vi "Compile ESTTL.vi"(8 "error in (no error)":errorcluster, 10 "PB-01 Compiled Data":T1, 11 "Device Item Ref in":T4 format="%.0x") -> (0 "error out":errorcluster, 2 "PB-01 Compiled Data out":T1, 3 "Device Item Ref out":T4 format="%.0x")   [LabVIEW 2015, in "DCM System Explorer.lvlib"]
uses:
  DCM System Explorer.lvlib
  <vilib>/NI Veristand/Custom Device API/Custom Device Item Ref.ctl
  Shared/Types/ESTTL Setup Indexes.ctl
  Shared/Types/PB-01.ctl
  <vilib>/Powertrain Controls/Device Drivers/VR-Hall/RevC/Real-Time/Support/Vr_Hall_mode_control_revc.ctl
  Shared/DCM Constants and GUIDs.vi
  <vilib>/NI Veristand/Custom Device Tools/Custom Device Utility Library/NI VeriStand - Search for Item by GUID.vi
  <vilib>/NI Veristand/Custom Device Tools/Custom Device Utility Library/Custom Device Utility Library.lvlib
  DCM Shared.lvlib
  <vilib>/NI VeriStand/Custom Device API/Custom Device API.lvlib
panel:
  in  "Command":T2[](array[typedef])=[{"Mode"=-1, "Polarity"=-1, "Frequency [Hz]"=-1, "Duty Cycle [%]"=-1, "TDC Offset [CAD]"=-1, "Window Start [DBTDC]"=-1, "Window End [DBTDC]"=0, "Angles"=[{"Enable"=0, "Location [DBTDC]"=0, "Duration [s]"=0}, {"Enable"=0, "Location [DBTDC]"=0, "Duration [s]"=0}, {"Enable"=0, "Location [DBTDC]"=0, "Duration [s]"=0}, {"Enable"=0, "Location [DBTDC]"=0, "Duration [s]"=0}], "Skip Fire"=-1, "Skip Fire Index"=-1}, {"Mode"=-1, "Polarity"=-1, "Frequency [Hz]"=-1, "Duty Cycle [%]"=-1, "TDC Offset [CAD]"=-1, "Window Start [DBTDC]"=-1, "Window End [DBTDC]"=0, "Angles"=[{"Enable"=0, "Location [DBTDC]"=0, "Duration [s]"=0}, {"Enable"=0, "Location [DBTDC]"=0, "Duration [s]"=0}, {"Enable"=0, "Location [DBTDC]"=0, "Duration [s]"=0}, {"Enable"=0, "Location [DBTDC]"=0, "Duration [s]"=0}], "Skip Fire"=-1, "Skip Fire Index"=-1}, {"Mode"=-1, "Polarity"=-1, "Frequency [Hz]"=-1, "Duty Cycle [%]"=-1, "TDC Offset [CAD]"=-1, "Window Start [DBTDC]"=-1, "Window End [DBTDC]"=0, "Angles"=[{"Enable"=0, "Location [DBTDC]"=0, "Duration [s]"=0}, {"Enable"=0, "Location [DBTDC]"=0, "Duration [s]"=0}, {"Enable"=0, "Location [DBTDC]"=0, "Duration [s]"=0}, {"Enable"=0, "Location [DBTDC]"=0, "Duration [s]"=0}], "Skip Fire"=-1, "Skip Fire Index"=-1}, {"Mode"=-1, "Polarity"=-1, "Frequency [Hz]"=-1, "Duty Cycle [%]"=-1, "TDC Offset [CAD]"=-1, "Window Start [DBTDC]"=-1, "Window End [DBTDC]"=0, "Angles"=[{"Enable"=0, "Location [DBTDC]"=0, "Duration [s]"=0}, {"Enable"=0, "Location [DBTDC]"=0, "Duration [s]"=0}, {"Enable"=0, "Location [DBTDC]"=0, "Duration [s]"=0}, {"Enable"=0, "Location [DBTDC]"=0, "Duration [s]"=0}], "Skip Fire"=-1, "Skip Fire Index"=-1}, {"Mode"=-1, "Polarity"=-1, "Frequency [Hz]"=-1, "Duty Cycle [%]"=-1, "TDC Offset [CAD]"=-1, "Window Start [DBTDC]"=-1, "Window End [DBTDC]"=0, "Angles"=[{"Enable"=0, "Location [DBTDC]"=0, "Duration [s]"=0}, {"Enable"=0, "Location [DBTDC]"=0, "Duration [s]"=0}, {"Enable"=0, "Location [DBTDC]"=0, "Duration [s]"=0}, {"Enable"=0, "Location [DBTDC]"=0, "Duration [s]"=0}], "Skip Fire"=-1, "Skip Fire Index"=-1}, {"Mode"=-1, "Polarity"=-1, "Frequency [Hz]"=-1, "Duty Cycle [%]"=-1, "TDC Offset [CAD]"=-1, "Window Start [DBTDC]"=-1, "Window End [DBTDC]"=0, "Angles"=[{"Enable"=0, "Location [DBTDC]"=0, "Duration [s]"=0}, {"Enable"=0, "Location [DBTDC]"=0, "Duration [s]"=0}, {"Enable"=0, "Location [DBTDC]"=0, "Duration [s]"=0}, {"Enable"=0, "Location [DBTDC]"=0, "Duration [s]"=0}], "Skip Fire"=-1, "Skip Fire Index"=-1}, {"Mode"=-1, "Polarity"=-1, "Frequency [Hz]"=-1, "Duty Cycle [%]"=-1, "TDC Offset [CAD]"=-1, "Window Start [DBTDC]"=-1, "Window End [DBTDC]"=0, "Angles"=[{"Enable"=0, "Location [DBTDC]"=0, "Duration [s]"=0}, {"Enable"=0, "Location [DBTDC]"=0, "Duration [s]"=0}, {"Enable"=0, "Location [DBTDC]"=0, "Duration [s]"=0}, {"Enable"=0, "Location [DBTDC]"=0, "Duration [s]"=0}], "Skip Fire"=-1, "Skip Fire Index"=-1}, {"Mode"=-1, "Polarity"=-1, "Frequency [Hz]"=-1, "Duty Cycle [%]"=-1, "TDC Offset [CAD]"=-1, "Window Start [DBTDC]"=-1, "Window End [DBTDC]"=0, "Angles"=[{"Enable"=0, "Location [DBTDC]"=0, "Duration [s]"=0}, {"Enable"=0, "Location [DBTDC]"=0, "Duration [s]"=0}, {"Enable"=0, "Location [DBTDC]"=0, "Duration [s]"=0}, {"Enable"=0, "Location [DBTDC]"=0, "Duration [s]"=0}], "Skip Fire"=-1, "Skip Fire Index"=-1}, {"Mode"=-1, "Polarity"=-1, "Frequency [Hz]"=-1, "Duty Cycle [%]"=-1, "TDC Offset [CAD]"=-1, "Window Start [DBTDC]"=-1, "Window End [DBTDC]"=0, "Angles"=[{"Enable"=0, "Location [DBTDC]"=0, "Duration [s]"=0}, {"Enable"=0, "Location [DBTDC]"=0, "Duration [s]"=0}, {"Enable"=0, "Location [DBTDC]"=0, "Duration [s]"=0}, {"Enable"=0, "Location [DBTDC]"=0, "Duration [s]"=0}], "Skip Fire"=-1, "Skip Fire Index"=-1}, {"Mode"=-1, "Polarity"=-1, "Frequency [Hz]"=-1, "Duty Cycle [%]"=-1, "TDC Offset [CAD]"=-1, "Window Start [DBTDC]"=-1, "Window End [DBTDC]"=0, "Angles"=[{"Enable"=0, "Location [DBTDC]"=0, "Duration [s]"=0}, {"Enable"=0, "Location [DBTDC]"=0, "Duration [s]"=0}, {"Enable"=0, "Location [DBTDC]"=0, "Duration [s]"=0}, {"Enable"=0, "Location [DBTDC]"=0, "Duration [s]"=0}], "Skip Fire"=-1, "Skip Fire Index"=-1}, {"Mode"=-1, "Polarity"=-1, "Frequency [Hz]"=-1, "Duty Cycle [%]"=-1, "TDC Offset [CAD]"=-1, "Window Start [DBTDC]"=-1, "Window End [DBTDC]"=0, "Angles"=[{"Enable"=0, "Location [DBTDC]"=0, "Duration [s]"=0}, {"Enable"=0, "Location [DBTDC]"=0, "Duration [s]"=0}, {"Enable"=0, "Location [DBTDC]"=0, "Duration [s]"=0}, {"Enable"=0, "Location [DBTDC]"=0, "Duration [s]"=0}], "Skip Fire"=-1, "Skip Fire Index"=-1}, {"Mode"=-1, "Polarity"=-1, "Frequency [Hz]"=-1, "Duty Cycle [%]"=-1, "TDC Offset [CAD]"=-1, "Window Start [DBTDC]"=-1, "Window End [DBTDC]"=0, "Angles"=[{"Enable"=0, "Location [DBTDC]"=0, "Duration [s]"=0}, {"Enable"=0, "Location [DBTDC]"=0, "Duration [s]"=0}, {"Enable"=0, "Location [DBTDC]"=0, "Duration [s]"=0}, {"Enable"=0, "Location [DBTDC]"=0, "Duration [s]"=0}], "Skip Fire"=-1, "Skip Fire Index"=-1}, {"Mode"=-1, "Polarity"=-1, "Frequency [Hz]"=-1, "Duty Cycle [%]"=-1, "TDC Offset [CAD]"=-1, "Window Start [DBTDC]"=-1, "Window End [DBTDC]"=0, "Angles"=[{"Enable"=0, "Location [DBTDC]"=0, "Duration [s]"=0}, {"Enable"=0, "Location [DBTDC]"=0, "Duration [s]"=0}, {"Enable"=0, "Location [DBTDC]"=0, "Duration [s]"=0}, {"Enable"=0, "Location [DBTDC]"=0, "Duration [s]"=0}], "Skip Fire"=-1, "Skip Fire Index"=-1}, {"Mode"=-1, "Polarity"=-1, "Frequency [Hz]"=-1, "Duty Cycle [%]"=-1, "TDC Offset [CAD]"=-1, "Window Start [DBTDC]"=-1, "Window End [DBTDC]"=0, "Angles"=[{"Enable"=0, "Location [DBTDC]"=0, "Duration [s]"=0}, {"Enable"=0, "Location [DBTDC]"=0, "Duration [s]"=0}, {"Enable"=0, "Location [DBTDC]"=0, "Duration [s]"=0}, {"Enable"=0, "Location [DBTDC]"=0, "Duration [s]"=0}], "Skip Fire"=-1, "Skip Fire Index"=-1}, {"Mode"=-1, "Polarity"=-1, "Frequency [Hz]"=-1, "Duty Cycle [%]"=-1, "TDC Offset [CAD]"=-1, "Window Start [DBTDC]"=-1, "Window End [DBTDC]"=0, "Angles"=[{"Enable"=0, "Location [DBTDC]"=0, "Duration [s]"=0}, {"Enable"=0, "Location [DBTDC]"=0, "Duration [s]"=0}, {"Enable"=0, "Location [DBTDC]"=0, "Duration [s]"=0}, {"Enable"=0, "Location [DBTDC]"=0, "Duration [s]"=0}], "Skip Fire"=-1, "Skip Fire Index"=-1}, {"Mode"=-1, "Polarity"=-1, "Frequency [Hz]"=-1, "Duty Cycle [%]"=-1, "TDC Offset [CAD]"=-1, "Window Start [DBTDC]"=-1, "Window End [DBTDC]"=0, "Angles"=[{"Enable"=0, "Location [DBTDC]"=0, "Duration [s]"=0}, {"Enable"=0, "Location [DBTDC]"=0, "Duration [s]"=0}, {"Enable"=0, "Location [DBTDC]"=0, "Duration [s]"=0}, {"Enable"=0, "Location [DBTDC]"=0, "Duration [s]"=0}], "Skip Fire"=-1, "Skip Fire Index"=-1}]
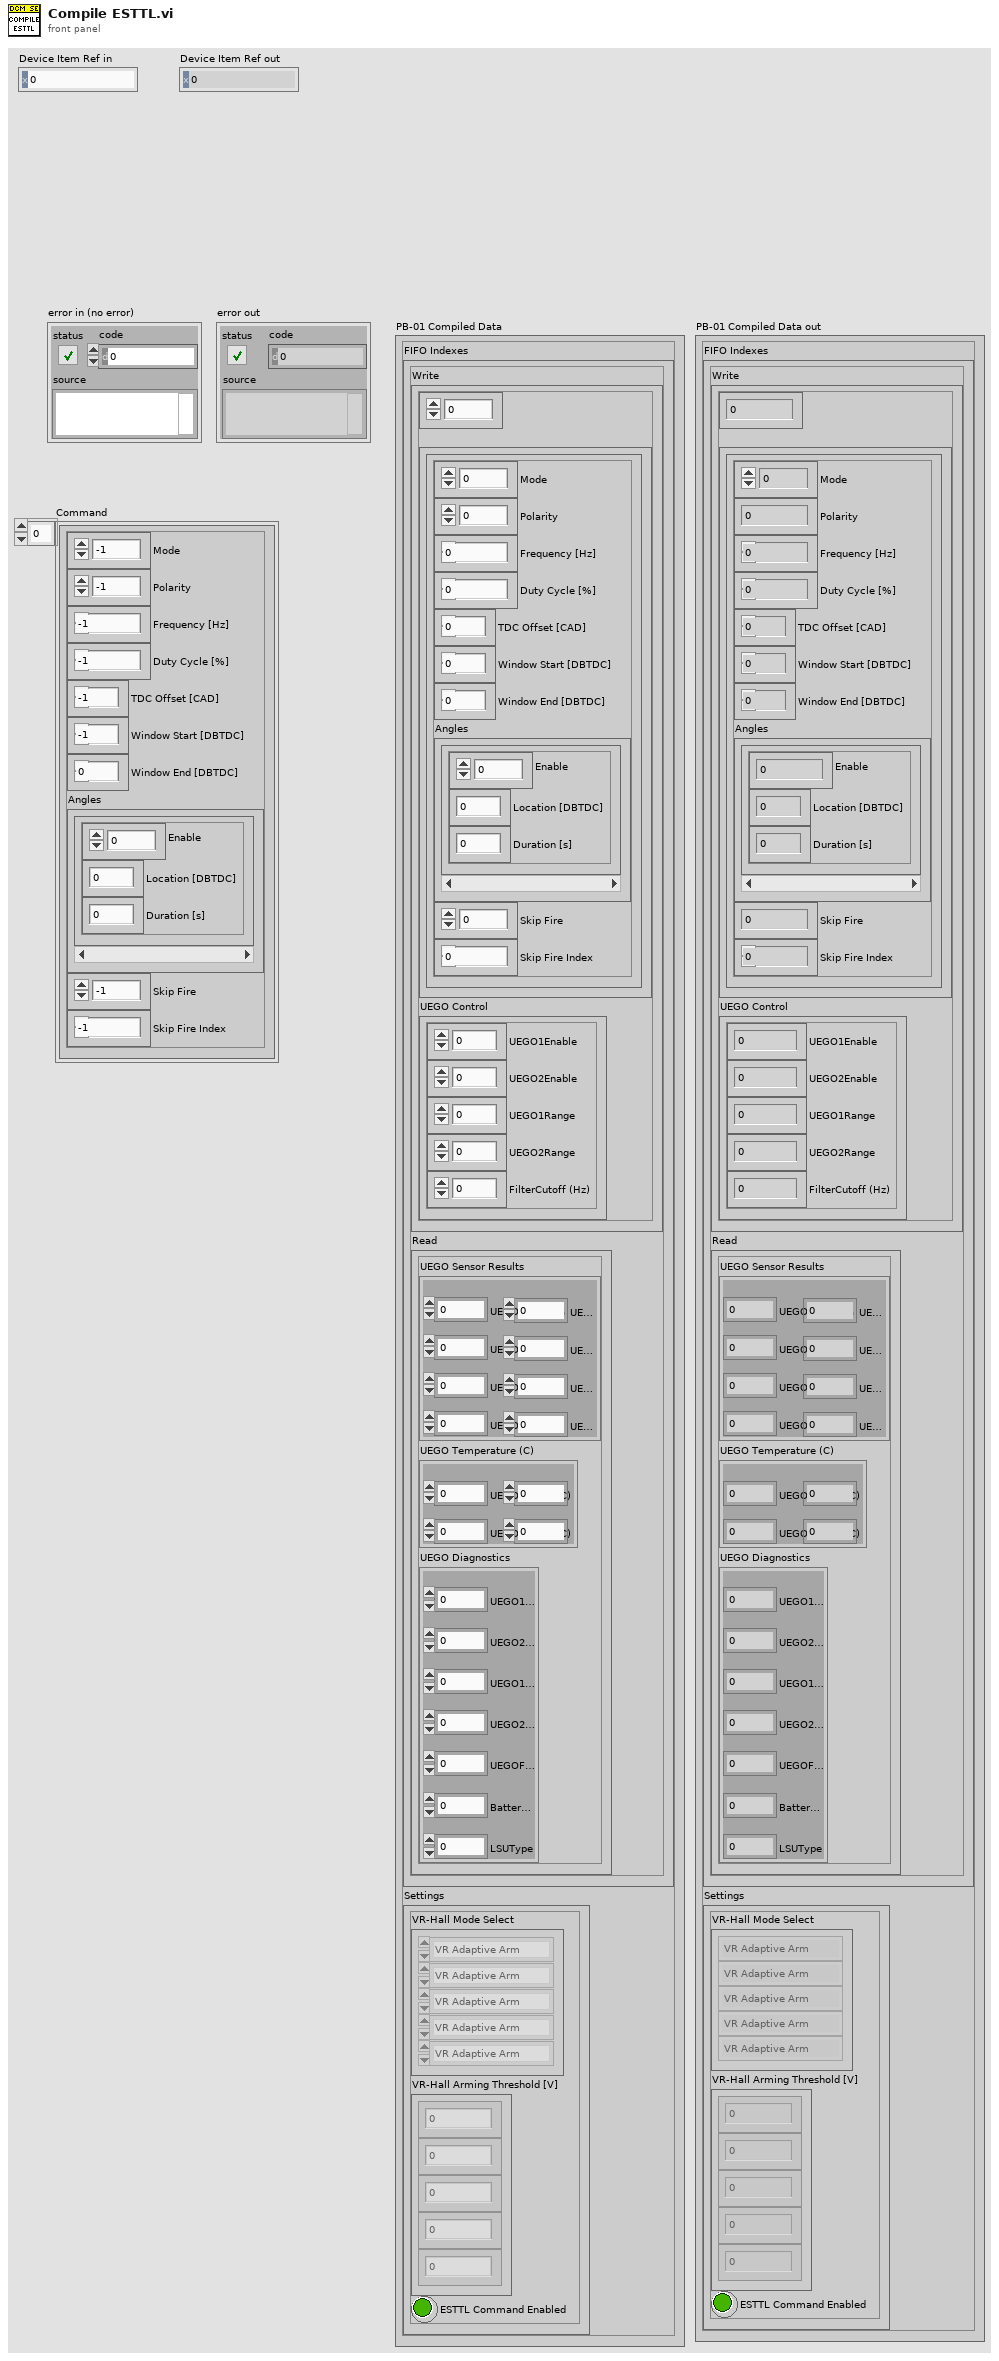
[diagram p1: front panel]
types:
  T1 = typedef "DCM Shared.lvlib/PB-01.ctl" = cluster{"FIFO Indexes":cluster{"Write":cluster{"Clear Faults":i32, "ESTTL Setup":T2[], "UEGO Control":cluster{"UEGO1Enable":i32, "UEGO2Enable":i32, "UEGO1Range":i32, "UEGO2Range":i32, "FilterCutoff (Hz)":i32}}, "Read":cluster{"UEGO Sensor Results":cluster{"UEGO1Lambda":i32, "UEGO1Phi":i32, "UEGO1AFRatio":i32, "UEGO1Ip (mA)":i32, "UEGO2Lambda":i32, "UEGO2Phi":i32, "UEGO2AFRatio":i32, "UEGO2Ip (mA)":i32}, "UEGO Temperature (C)":cluster{"UEGO1Temp (C)":i32, "UEGO2Temp (C)":i32, "UEGO1Hot":i32, "UEGO2Hot":i32}, "UEGO Diagnostics":cluster{"UEGO1SensorFault":i32, "UEGO2SensorFault":i32, "UEGO1HeaterFault":i32, "UEGO2HeaterFault":i32, "UEGOFuseStatus":i32, "Battery (V)":i32, "LSUType":i32}}}, "Settings":cluster{"VR-Hall Mode Select":T3[], "VR-Hall Arming Threshold [V]":dbl[], "ESTTL Command Enabled":bool}}
  T2 = typedef "DCM Shared.lvlib/ESTTL Setup Indexes.ctl" = cluster{"Mode":i32, "Polarity":i32, "Frequency [Hz]":i32, "Duty Cycle [%]":i32, "TDC Offset [CAD]":i32, "Window Start [DBTDC]":i32, "Window End [DBTDC]":i32, "Angles":cluster{"Enable":i32, "Location [DBTDC]":i32, "Duration [s]":i32}[], "Skip Fire":i32, "Skip Fire Index":i32}
  T3 = typedef "Vr_Hall_mode_control_revc.ctl" = enum32{"VR Adaptive Arm", "VR Manual Arm", "Hall", "Hall w/ Pull-up"}
  T4 = typedef "Custom Device API.lvlib/Custom Device Item Ref.ctl" = u64
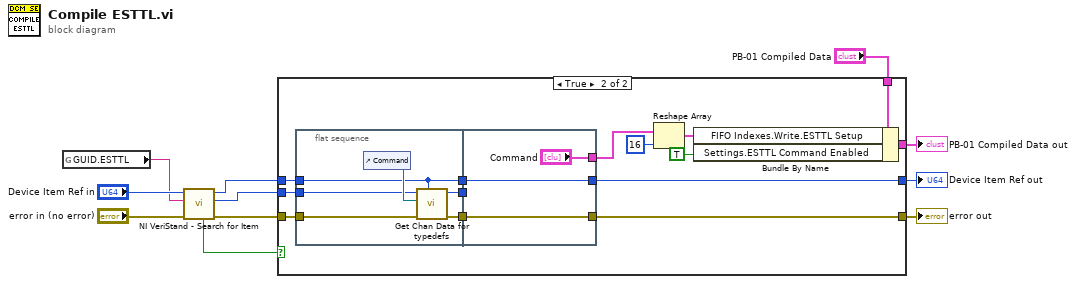
[diagram p0: block diagram]
diagram:
  n1 = global read "DCM Constants and GUIDs.vi" "GUID.ESTTL"() -> (w9:string)
  n2 = call-poly <vilib>:"NI VeriStand - Search for Item.vi"("error in"="error in (no error)", "Item GUID"=w9, "Section Ref in"="Device Item Ref in") -> ("error out"=w8:errorcluster, "Item Ref"=w7:T4, "Section Ref out"=w6:T4, "Found"=w1:bool)  [unwired: 5 in]
  n3 = case shown="True" w1 {
    tunnel: w8 -> [w12 w25]
    tunnel: w7 -> [_ w24]
    tunnel: w6 -> [w13 w23]
    tunnel: [w14 w21] -> w5
    tunnel: "PB-01 Compiled Data" -> [w14 w20]
    tunnel: [w13 w17] -> w3
    tunnel: [w12 w16] -> w2
    frame False {
    }
    frame True {
      n4 = flat-sequence {
        tunnel: w25 -> [w34]
        tunnel: w24 -> [w31]
        tunnel: [w33] -> w28
        tunnel: [w30] -> w27
        tunnel: w23 -> [w29]
        tunnel: [w29] -> w26
        tunnel: [w37] -> w16
        tunnel: w28 -> [w37]
        tunnel: w27 -> [_]
        tunnel: ["Command"] -> w19
        tunnel: w26 -> [w36]
        tunnel: [w36] -> w17
        frame #0 {
          n5 = control-ref of="Command"() -> (w32:refnum<vi>)
          n6 = call "Get Chan Data for typedefs.vi"("Custom Device Ref"=w29, "error in"=w34, "Ctl Ref"=w32, "Section Ref in"=w31) -> ("error out"=w33:errorcluster, "Section Ref out"=w30:T4)  [unwired: 6 in]
        }
        frame #1 {
        }
      }
      n7 = Reshape Array(w19, 16 ("dimension size")) -> (w18:T2[])
      n8 = Bundle By Name(cluster=w20, "FIFO Indexes.Write.ESTTL Setup"=w18, "Settings.ESTTL Command Enabled"=TRUE) -> (w21:T1)
    }
  }
  "error out" <- w2
  "Device Item Ref out" <- w3
  "PB-01 Compiled Data out" <- w5
